vi "Waveform_Append and Resize Allocated.vi"(8 "Error":errorcluster, 9 "Append":T1, 11 "Waveform":T1) -> (0 "Error Out":errorcluster, 3 "Waveform Out":T1, 5 "Offset Out":i32)   [LabVIEW 2025]
uses:
  Universal Controls/Waveform_Data.ctl
  Universal Controls/Read Write Button.ctl
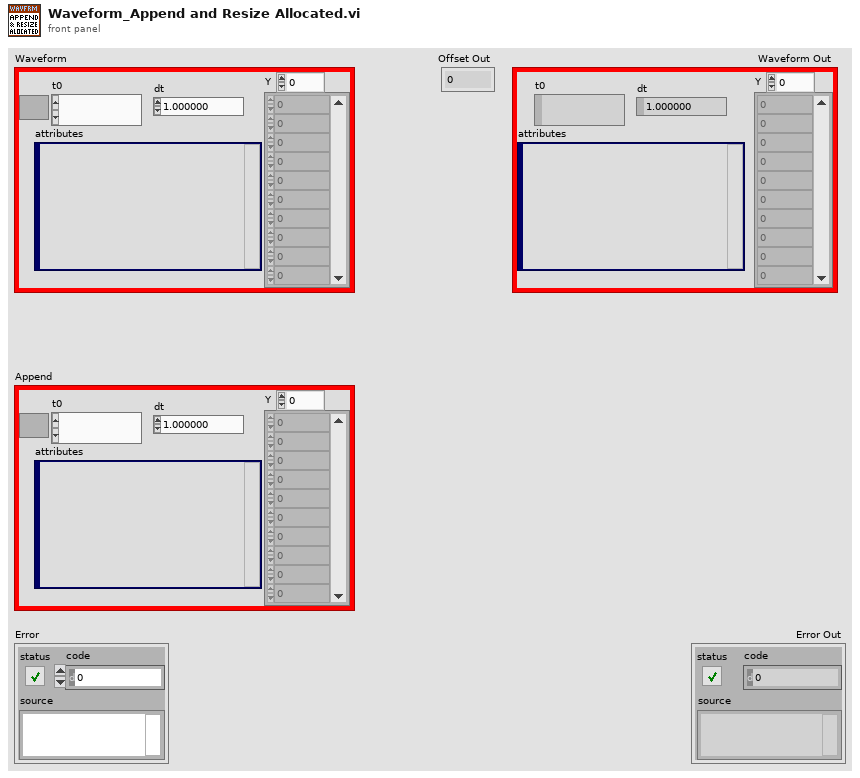
[diagram p1: front panel]
types:
  T1 = typedef "Waveform_Data.ctl" = waveform(dbl)
  T2 = typedef "Read Write Button.ctl" = bool
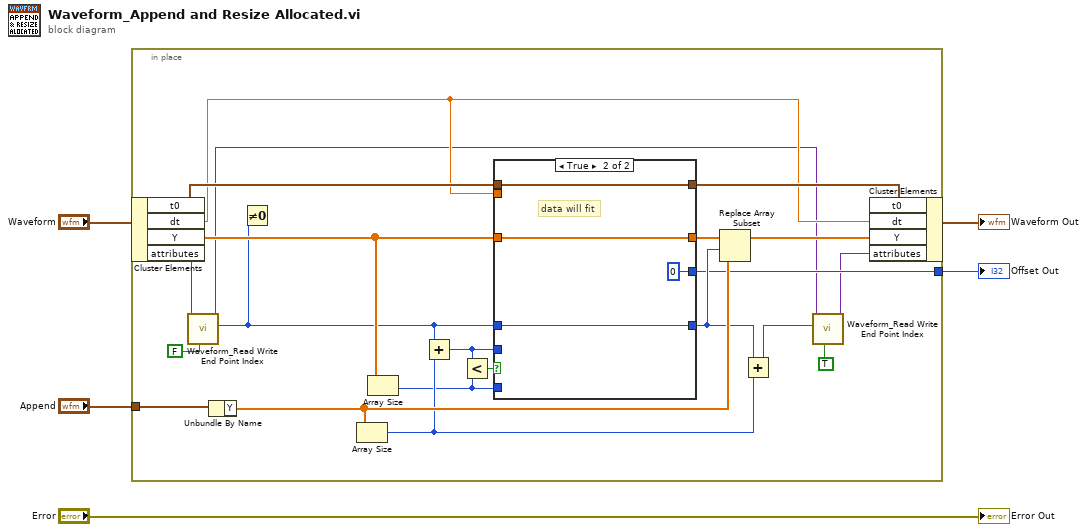
[diagram p0: block diagram]
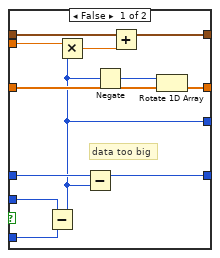
[diagram p2: hidden frame]
diagram:
  n1 = in-place {
    in-place-border: "Append" -> [w26]
    in-place-border: [w18] -> w3
    n2 = in-place-cluster #1("Waveform") -> ("t0"=w17:timestamp, "dt"=w8:dbl, "Y"=w24:dbl[], "attributes"=w13:variant)
    n3 = call "Waveform_Read Write End Point Index.vi"("Read(f)\nWrite(t)"=T2 FALSE ("Read(f)\nWrite(t)"), "Waveform Attributes"=w13) -> ("End Point Out"=w6:i32, "Waveform Attributes Out"=w7:variant)  [unwired: 6 in, 2 out]
    n4 = Unbundle By Name(w26) -> ("Y"=w22:dbl[])
    n5 = Not Equal To 0?(x=w6) -> ()  [unwired: 1 out]
    n6 = Array Size(array=w22) -> (size(s)=w20:i32)
    n7 = Array Size(array=w24) -> (size(s)=w14:i32)
    n8 = Add(x=w6, y=w20) -> (x+y=w15:i32)
    n9 = Less?(x=w15, y=w14) -> (x < y?=w25:bool)
    n10 = case shown="True" w25 {
      tunnel: w15 -> [w37 _]
      tunnel: w14 -> [w38 _]
      tunnel: w6 -> [w35 w42]
      tunnel: w24 -> [w36 w41]
      tunnel: [w34 w41] -> w23
      tunnel: [w33 w42] -> w19
      tunnel: [w31 0] -> w18
      tunnel: w17 -> [w32 w40]
      tunnel: [w29 w40] -> w16
      tunnel: w8 -> [w30 _]
      frame False {
        # "data too big"
        n11 = Subtract(x=w37, y=w38) -> (x-y=w31:i32)
        n12 = Multiply(x=w30, y=w31) -> (x*y=w28:dbl)
        n13 = Subtract(x=w35, y=w31) -> (x-y=w33:i32)
        n14 = Negate(x=w31) -> (-x=w27:i32)
        n15 = Add(x=w32, y=w28) -> (x+y=w29:timestamp)
        n16 = Rotate 1D Array(1:w36, 2:w27) -> (0:w34:dbl[])
      }
      frame True {
        # "data will fit"
      }
    }
    n17 = Replace Array Subset(array=w23, new element=w22, index=w19) -> (w21:dbl[])
    n18 = Add(x=w19, y=w20) -> (x+y=w9:i32)
    n19 = call "Waveform_Read Write End Point Index.vi"("Read(f)\nWrite(t)"=T2 TRUE ("Read(f)\nWrite(t)"), "End Point"=w9, "Waveform Attributes"=w7) -> ("Waveform Attributes Out"=w12:variant)  [unwired: 5 in, 3 out]
    n20 = in-place-cluster #1("t0"=w16, "dt"=w8, "Y"=w21, "attributes"=w12) -> (→"Waveform Out":T1)
  }
  "Offset Out" <- w3
  "Error Out" <- "Error"
